vi "DSF.Engine.Transfer Group.Retrieve from FIFO.vi"(8 "error in (no error)":errorcluster, 10 "expected iteration":u64, 11 "Transfer Group in":refnum<class "DSF.Engine.Transfer Group.lvclass">) -> (0 "error out":errorcluster, 2 "iteration valid?":bool, 3 "Transfer Group out":refnum<class "DSF.Engine.Transfer Group.lvclass">)   [LabVIEW 2017, in "DSF.Engine.lvlib" / "DSF.Engine.Transfer Group.lvclass"]
uses:
  DSF.Engine.Transfer Group.lvclass
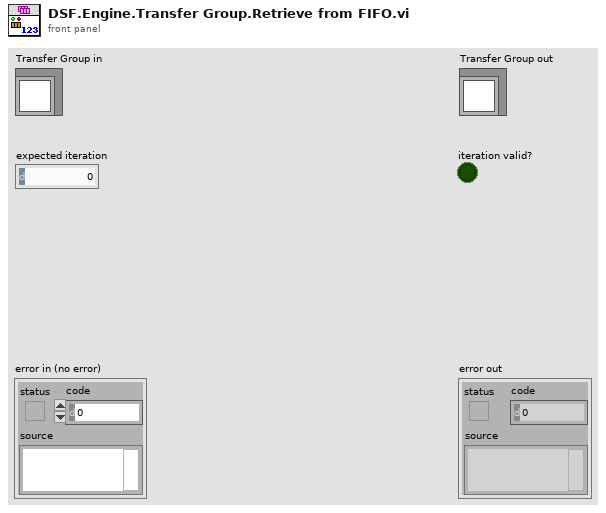
[diagram p1: front panel]
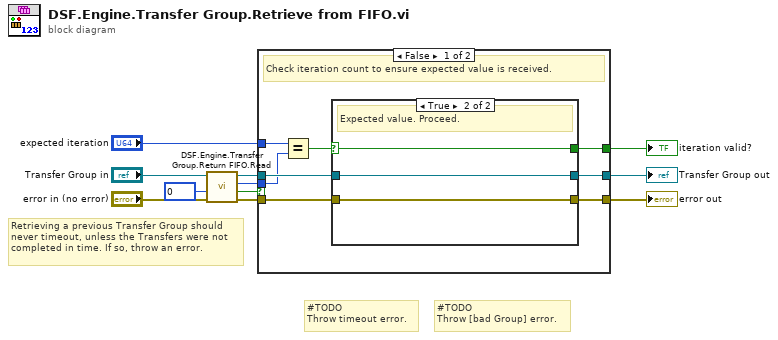
[diagram p0: block diagram]
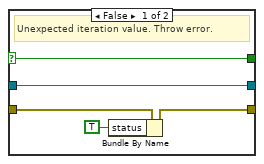
[diagram p2: hidden frame]
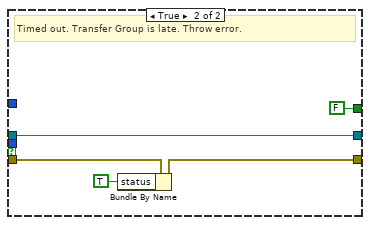
[diagram p3: hidden frame]
diagram:
  # "#TODO\nThrow [bad Group] error."
  # "#TODO\nThrow timeout error."
  # "Retrieving a previous Transfer Group should never timeout, unless the Transfers were not completed in time. If so, throw an error."
  n1 = call "DSF.Engine.Transfer Group.Return FIFO.Read.vi"("error in (no error)"="error in (no error)", "timeout in ms (0)"=0, "Transfer Group in"="Transfer Group in") -> ("error out"=w10:errorcluster, "timed out?"=w9:bool, "Transfer Group iteration"=w7:u64, "Transfer Group out"=w8:refnum<class "DSF.Engine.Transfer Group.lvclass">)  [unwired: 5 in]
  n2 = case shown="False" w9 {
    tunnel: w10 -> [w15 w32]
    tunnel: w8 -> [w17 w29]
    tunnel: w7 -> [w13 _]
    tunnel: "expected iteration" -> [w19 _]
    tunnel: [w14 w31] -> w2
    tunnel: [w16 w29] -> w3
    tunnel: [w12 FALSE] -> w1
    frame False {
      # "Check iteration count to ensure expected value is received."
      n3 = Equal?(x=w19, y=w13) -> (x = y?=w18:bool)
      n4 = case shown="True" w18 {
        selector: w18 -> [w20 w25]
        tunnel: w17 -> [w24 w27]
        tunnel: [w24 w27] -> w16
        tunnel: w15 -> [w23 w26]
        tunnel: [w22 w26] -> w14
        tunnel: [w20 w25] -> w12
        frame False {
          # "Unexpected iteration value. Throw error."
          n5 = Bundle By Name(cluster=w23, "status"=TRUE) -> (w22:errorcluster)
        }
        frame True {
          # "Expected value. Proceed."
        }
      }
    }
    frame True {
      # "Timed out. Transfer Group is late. Throw error."
      n6 = Bundle By Name(cluster=w32, "status"=TRUE) -> (w31:errorcluster)
    }
  }
  "error out" <- w2
  "Transfer Group out" <- w3
  "iteration valid?" <- w1
